vi "Get Failure Action Event References.vi"(8 "error in (no error)":errorcluster, 11 "Assert Name":string) -> (0 "error out":errorcluster, 2 "Event Registration Refnum":refnum<event-registration>, 3 "Failure Action Change Event":refnum<user-event>)   [LabVIEW 2016, in "AssertEngine.lvlib"]
doc: "Gets the event references (either by creating if it doesn't previously exist or by recovering it if it does) to be used for detecting a change in failure action."
uses:
  AssertEngine.lvlib
  Failure Action Lookup Table TypeDef.ctl
  Failure Action FGV TypeDef.ctl
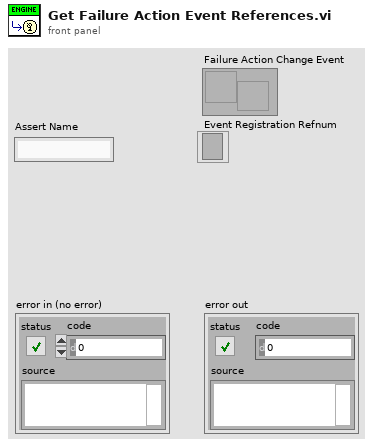
[diagram p1: front panel]
types:
  T1 = typedef "AssertEngine.lvlib/Failure Action Lookup Table TypeDef.ctl" = cluster{"Assert Name List":string[], "Event Array":T2[]}
  T2 = typedef "AssertEngine.lvlib/Failure Action FGV TypeDef.ctl" = cluster{"Failure Action Change Event":refnum<user-event>, "Event Registration Refnum":refnum<event-registration>}
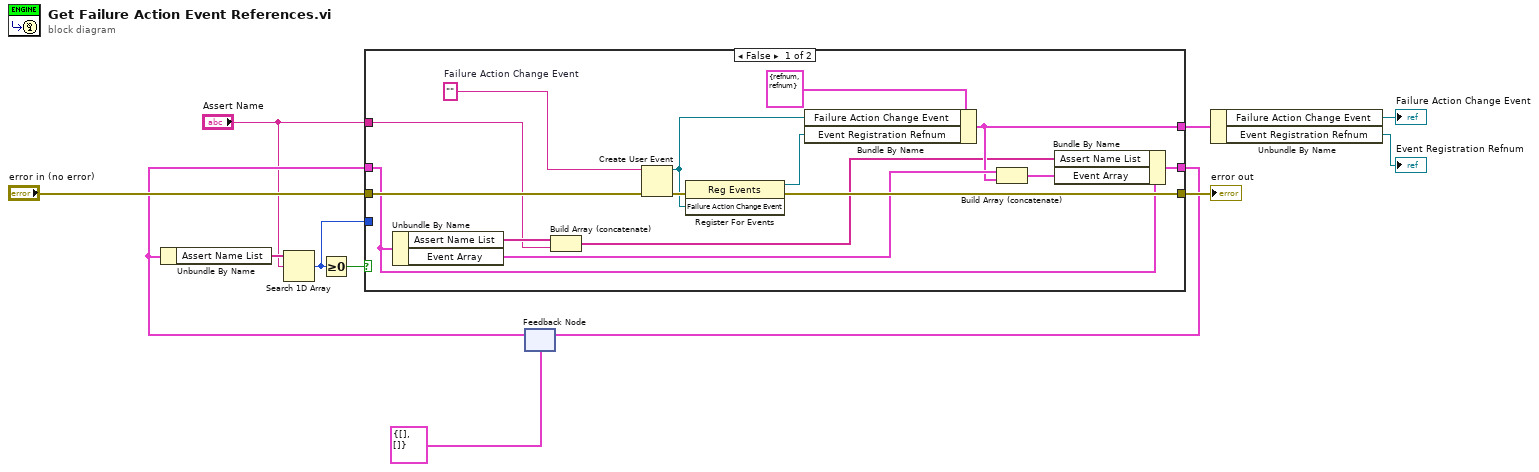
[diagram p0: block diagram]
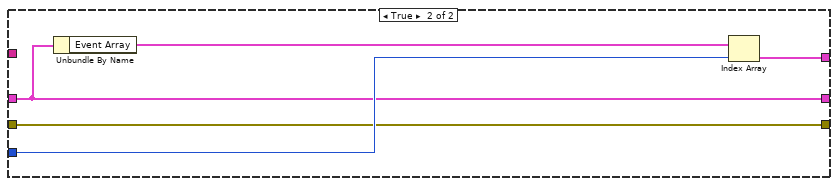
[diagram p2: hidden frame]
diagram:
  n1 = feedback #1(T1 {"Assert Name List"=[], "Event Array"=[]} ("Event Registration Lookup Table")) -> (w8:T1)
  n2 = Unbundle By Name(w8) -> ("Assert Name List"=w10:string[])
  n3 = Search 1D Array(1D array=w10, element="Assert Name") -> (index of element=w7:i32)  [unwired: 1 in]
  n4 = Greater Or Equal To 0?(x=w7) -> (x >= 0?=w9:bool)
  n5 = case shown="False" w9 {
    tunnel: [w27 w29] -> w12
    tunnel: "error in (no error)" -> [w26 w29]
    tunnel: w8 -> [w16 w28]
    tunnel: w7 -> [_ w31]
    tunnel: [w17 w30] -> w6
    tunnel: "Assert Name" -> [w19 _]
    tunnel: [w13 w28] -> w1
    frame False {
      w25 = ""  # Failure Action Change Event
      n6 = Unbundle By Name(w16) -> ("Assert Name List"=w20:string[], "Event Array"=w18:T2[])
      n7 = Build Array (concatenate)(w20, w19) -> (w15:string[])
      n8 = Create User Event(user event datatype=w25, error in=w26) -> (user event=w22:refnum<user-event>, error out=w24:errorcluster)
      n9 = register-events(error in=w24, w22) -> (reference out=w21:refnum<event-registration>, error out=w27:errorcluster)  [unwired: 1 in]
      n10 = Bundle By Name(cluster=T2 {"Failure Action Change Event"=refnum, "Event Registration Refnum"=refnum} ("Cluster"), "Failure Action Change Event"=w22, "Event Registration Refnum"=w21) -> (w17:T2)
      n11 = Build Array (concatenate)(w18, w17) -> (w14:T2[])
      n12 = Bundle By Name(cluster=w16, "Assert Name List"=w15, "Event Array"=w14) -> (w13:T1)
    }
    frame True {
      n13 = Unbundle By Name(w28) -> ("Event Array"=w32:T2[])
      n14 = Index Array(array=w32, index=w31) -> (element=w30:T2)
    }
  }
  "error out" <- w12
  n15 = feedback-in #1(w1) -> ()
  n16 = Unbundle By Name(w6) -> ("Failure Action Change Event"=→"Failure Action Change Event":refnum<user-event>, "Event Registration Refnum"=→"Event Registration Refnum":refnum<event-registration>)
